vi "load.vi"() -> (0 "calibration vol. [ml]":dbl=10670.0, 1 "humidity [%]":dbl, 2 "pressure [mbar]":dbl, 3 "temperature [°C]":dbl, 4 "pipette vol. [ml]":dbl=0.2148, 5 "CA-Name":string, 6 "additional vol. [ml]":dbl=11.0, 7 "canceled?":bool)   [LabVIEW 2013]
uses:
  Instance           1 12Saved   load .vi
  <vilib>/Utility/config.llb/Read Key (Double).vi
  <vilib>/Utility/config.llb/NI_LVConfig.lvlib
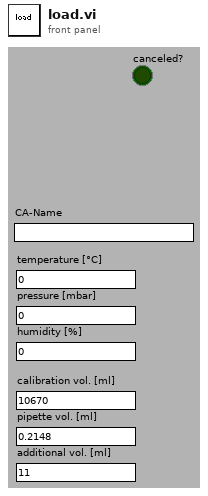
[diagram p1: front panel]
types:
  T1 = typedef "NI_LVConfig.lvlib/Config Data RefNum.ctl" = refnum<k1>
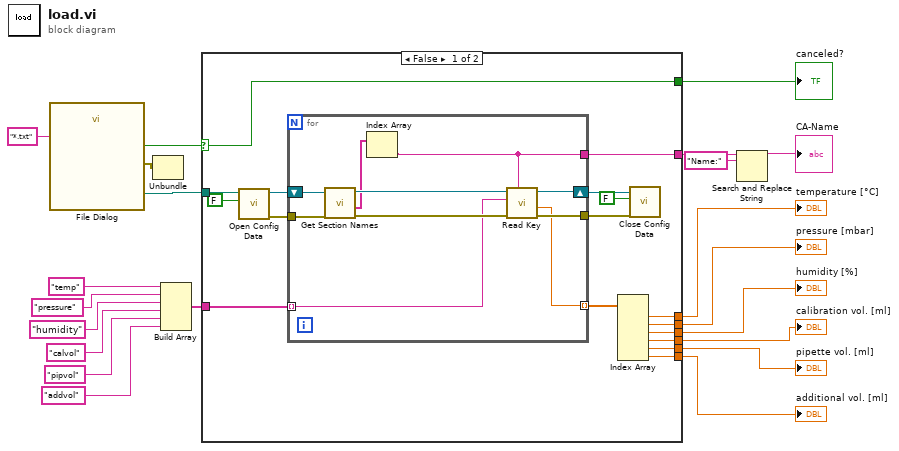
[diagram p0: block diagram]
diagram:
  n1 = call "File Dialog"("pattern (all files)"="*.txt") -> ("selected path"=w13:path, "cancelled"=w14:bool, "error out"=w1:errorcluster)  [unwired: 11 in, 1 out]
  n2 = Unbundle(w1) -> ()  [unwired: 3 out]
  n3 = Build Array("temp", "pressure", "humidity", "calvol", "pipvol", "addvol") -> (w15:string[])
  n4 = case shown="False" w14 {
    selector: w14 -> [w31 w49]
    tunnel: w15 -> [w36 _]
    tunnel: w13 -> [w34 _]
    tunnel: [w32 _] -> w4
    tunnel: [w31 w49] -> w11
    tunnel: [w29 _] -> w10
    tunnel: [w28 _] -> w9
    tunnel: [w27 _] -> w8
    tunnel: [w26 _] -> w7
    tunnel: [w25 _] -> w6
    tunnel: [w24 _] -> w5
    frame False {
      n5 = call <vilib>:"Open Config Data.vi"("create file if necessary (T)"=FALSE ("create file if necessary? (T)"), "configuration file path"=w34) -> ("error out"=w37:errorcluster, "refnum"=w38:T1)  [unwired: 7 in, 1 out]
      n6 = for {
        tunnel: w37 -> [w47]
        shift-right: [w44] -> w35
        shift-left: w38 -> [w48]
        tunnel: w36 -> [w41] mode=indexing
        tunnel: [w43] -> w33
        tunnel: [w39] -> w32
        tunnel: [w40] -> w30 mode=indexing
        n7 = call <vilib>:"Get Section Names.vi"("error in (no error)"=w47, "refnum"=w48) -> ("error out"=w46:errorcluster, "section names"=w42:string[], "refnum out"=w45:T1)  [unwired: 7 in]
        n8 = Index Array(array=w42) -> (element=w39:string)  [unwired: 1 in]
        n9 = call-poly <vilib>:"Read Key.vi"("section"=w39, "error in (no error)"=w46, "key"=w41, "refnum"=w45) -> ("error out"=w43:errorcluster, "value"=w40:dbl, "refnum out"=w44:T1)  [unwired: 4 in, 1 out]
      }
      n10 = Index Array(array=w30) -> (element #1=w29:dbl, element #2=w28:dbl, element #3=w27:dbl, element #4=w26:dbl, element #5=w25:dbl, element #6=w24:dbl)  [unwired: 6 in]
      n11 = call <vilib>:"Close Config Data.vi"("error in (no error)"=w33, "write file if changed (T)"=FALSE ("write configuration file? (T)"), "refnum"=w35) -> ()  [unwired: 7 in, 2 out]
    }
    frame True {
    }
  }
  "temperature [°C]" <- w10
  "pressure [mbar]" <- w9
  "humidity [%]" <- w8
  "calibration vol. [ml]" <- w7
  "pipette vol. [ml]" <- w6
  "additional vol. [ml]" <- w5
  "canceled?" <- w11
  n12 = Search and Replace String(input string=w4, search string="Name:") -> (result string=→"CA-Name":string)  [unwired: 6 in, 3 out]
